vi "OcsReadListCsv.vi"() -> ()   [LabVIEW 2011]
panel:
  out "Stop":bool
  in  "Start":dbl
  out "Sec2":dbl
  in  "popup":bool=TRUE
  out "Numeric":i32
  out "stripped path":path
  out "path":path
  out "element":i32
  out "array":string[][](array[string])
  out "Out":string
  out "Start Time":dbl
  out "Sec":dbl
  # "Revision.1 20220617"
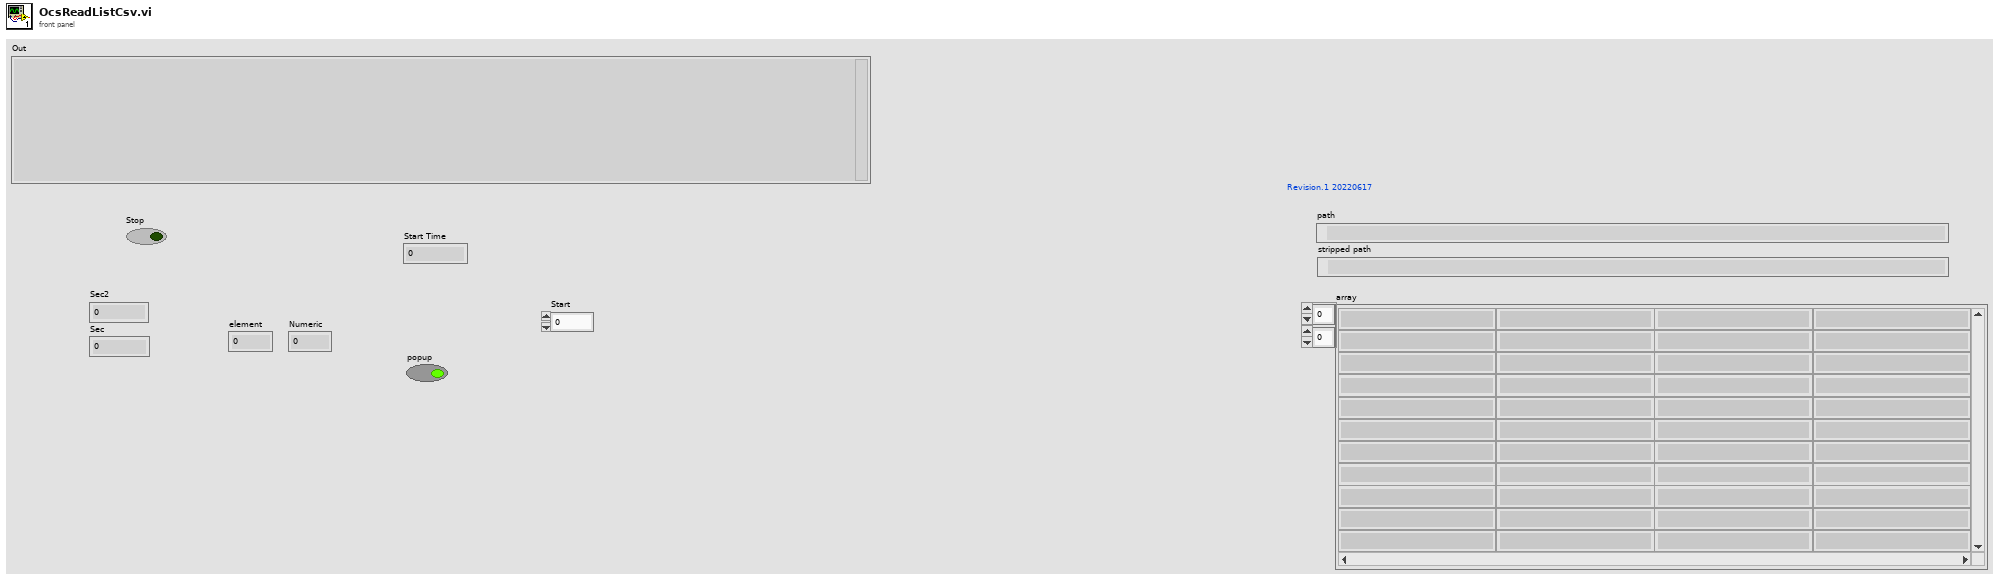
[diagram p1: front panel]
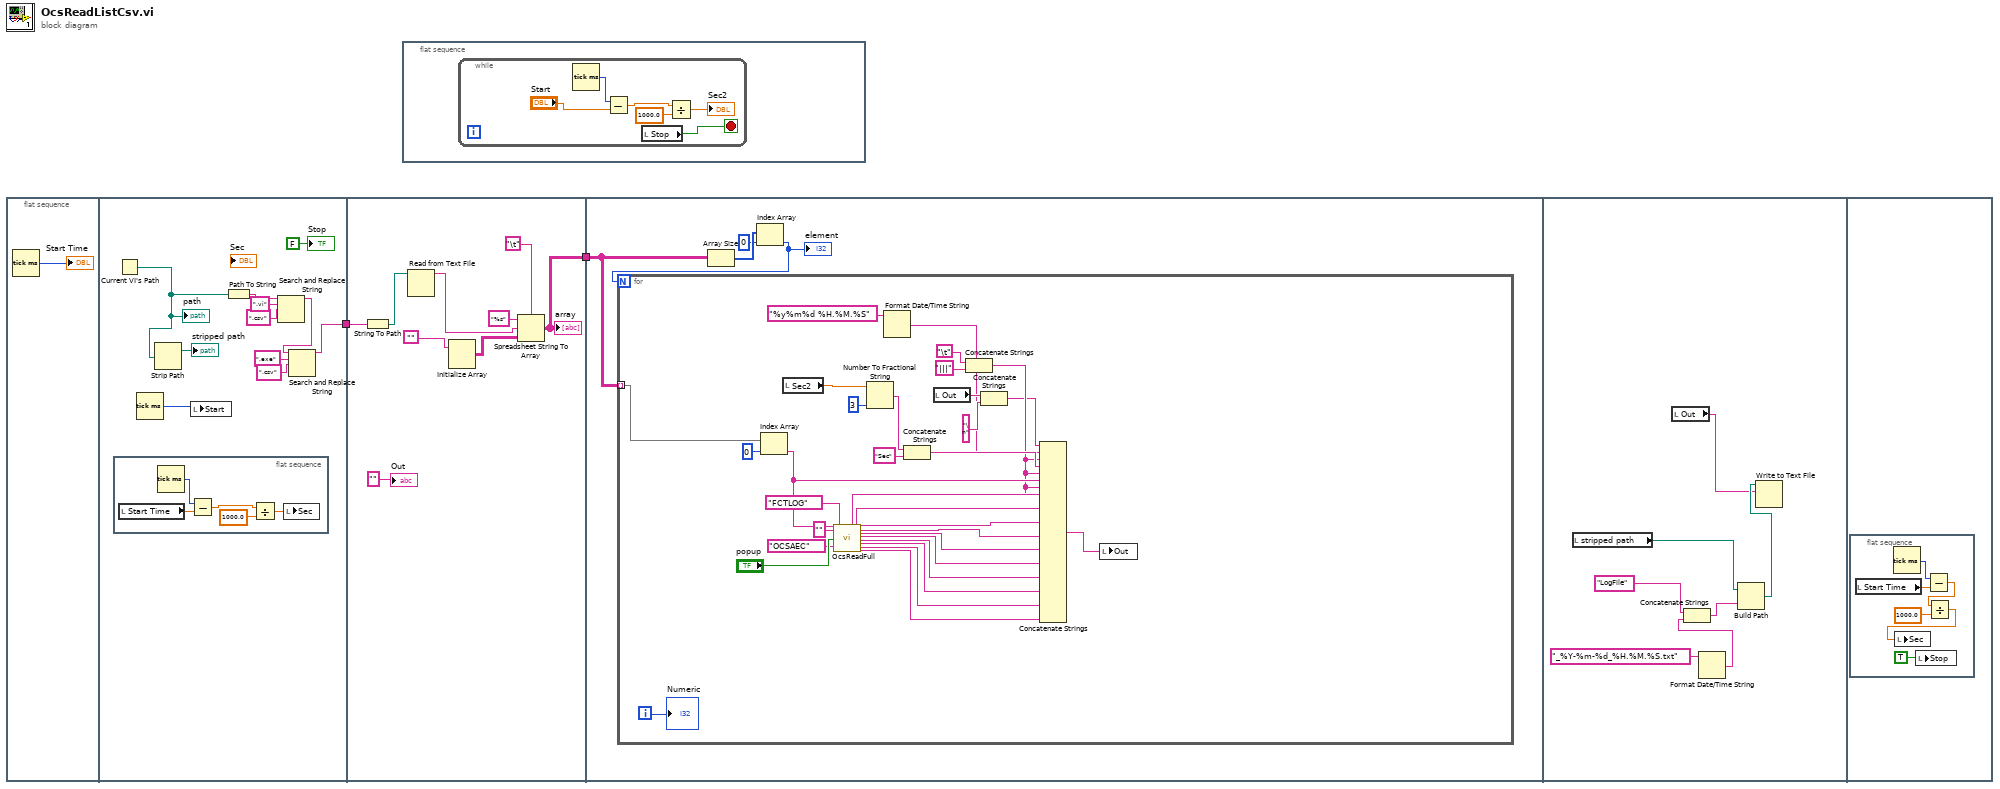
[diagram p0: block diagram]
diagram:
  n1 = flat-sequence {
    tunnel: [w6] -> w1
    tunnel: [w23] -> w2
    tunnel: w1 -> [w21]
    tunnel: w2 -> [w29]
    frame #0 {
      n2 = Tick Count (ms)() -> (millisecond timer value=→"Start Time":u32)
    }
    frame #1 {
      n3 = flat-sequence {
        frame #0 {
          n4 = local read "Start Time"() -> (w18:dbl)
          n5 = Tick Count (ms)() -> (millisecond timer value=w19:u32)
          n6 = Subtract(x=w19, y=w18) -> (x-y=w17:dbl)
          n7 = Divide(x=w17, y=1000.0) -> (x/y=w15:dbl)
          n8 = local write "Sec"(w15) -> ()
        }
      }
      n9 = Current VI's Path() -> (path=w13:path)
      "path" <- w13
      n10 = Tick Count (ms)() -> (millisecond timer value=w4:u32)
      n11 = Strip Path(path=w13) -> (stripped path=→"stripped path":path)  [unwired: 1 out]
      n12 = local write "Start"(w4) -> ()
      n13 = Path To String(path=w13) -> (string=w12:string)
      n14 = Search and Replace String(input string=w12, search string=".vi", replace string=".csv" ("replace string (\"\")")) -> (result string=w7:string)  [unwired: 5 in, 3 out]
      n15 = Search and Replace String(input string=w7, search string=".exe", replace string=".csv" ("replace string (\"\")")) -> (result string=w6:string)  [unwired: 5 in, 3 out]
      "Stop" <- FALSE ("Stop")
    }
    frame #2 {
      n16 = String To Path(string=w21) -> (path=w20:path)
      n17 = Read from Text File(file (use dialog)=w20) -> (text=w28:string)  [unwired: 3 in, 3 out]
      n18 = Initialize Array("") -> (w27:string[][])  [unwired: 2 in]
      n19 = Spreadsheet String To Array(delimiter (Tab)="\t", format string="%s", spreadsheet string=w28, array type (2D Dbl)=w27) -> (array=w23:string[][])
      "array" <- w23
      "Out" <- ""
    }
    frame #3 {
      n20 = Array Size(array=w29) -> (size(s)=w32:i32[])
      n21 = Index Array(array=w32, index=0) -> (element=w30:i32)
      "element" <- w30
      n22 = for {
        N: w30 -> [_]
        tunnel: w29 -> [w64] mode=indexing
        i -> [w46]
        n23 = Index Array(array=w64, index=0) -> (element=w42:string)
        n24 = local read "Sec2"() -> (w38:dbl)
        n25 = call "OcsReadFull.vi"("SN"=w42, "OPNAME Befor"="", "popup"="popup", "OcsThai"="OCSAEC", "TebelLogBefor"="FCTLOG") -> ("R1"=w60:string, "R2"=w59:string, "R3"=w58:string, "R4"=w57:string, "R5 SNPcb"=w56:string, "R6 SN BottomCase"=w55:string, "R7"=w54:string, "R8"=w53:string, "R9"=w52:string, "R10"=w51:string)  [unwired: 11 in, 2 out]
        n26 = Number To Fractional String(number=w38, precision (6)=i16 3) -> (F-format string=w37:string)  [unwired: 2 in]
        n27 = Format Date/Time String(time format string (%c)="%y%m%d %H.%M.%S") -> (date/time string=w34:string)  [unwired: 2 in]
        n28 = Concatenate Strings(w37, "Sec" ("string")) -> (w40:string)
        n29 = local read "Out"() -> (w44:string)
        n30 = Concatenate Strings("\t", "|||" ("string")) -> (w36:string)
        n31 = Concatenate Strings(w44, "\n" ("string")) -> (w33:string)
        n32 = Concatenate Strings(w33, w34, w36, w40, w36, w42, w36, w60, w36, w59, w36, w58, w36, w57, w36, w56, w36, w55, w36, w54, w36, w53, w36, w52, w36, w51) -> (w50:string)
        n33 = local write "Out"(w50) -> ()
        "Numeric" <- w46
      }
    }
    frame #4 {
      n34 = local read "stripped path"() -> (w65:path)
      n35 = local read "Out"() -> (w67:string)
      n36 = Format Date/Time String(time format string (%c)="_%Y-%m-%d_%H.%M.%S.txt") -> (date/time string=w69:string)  [unwired: 2 in]
      n37 = Concatenate Strings("LogFile" ("name or relative path"), w69) -> (w70:string)
      n38 = Build Path(base path=w65, name or relative path=w70) -> (appended path=w68:path)
      n39 = Write to Text File(file (use dialog)=w68, text=w67) -> ()  [unwired: 2 in, 3 out]
    }
    frame #5 {
      n40 = flat-sequence {
        frame #0 {
          n41 = local read "Start Time"() -> (w76:dbl)
          n42 = Tick Count (ms)() -> (millisecond timer value=w77:u32)
          n43 = local write "Stop"(TRUE ("Stop")) -> ()
          n44 = Subtract(x=w77, y=w76) -> (x-y=w75:dbl)
          n45 = Divide(x=w75, y=1000.0) -> (x/y=w73:dbl)
          n46 = local write "Sec"(w73) -> ()
        }
      }
    }
  }
  n47 = flat-sequence {
    frame #0 {
      n48 = while {
        stop <- w78 stop-if-true
        n49 = Tick Count (ms)() -> (millisecond timer value=w81:u32)
        n50 = Subtract(x=w81, y="Start") -> (x-y=w80:dbl)
        n51 = local read "Stop"() -> (w78:bool)
        n52 = Divide(x=w80, y=1000.0) -> (x/y=→"Sec2":dbl)
      }
    }
  }
